vi "Set Window Title.vi"(8 "error in (no error)":errorcluster, 11 "Actor in":refnum<class "Actor.lvclass">) -> (0 "error out":errorcluster)   [LabVIEW 2020, in "RTAF.lvlib" / "Actor.lvclass"]
uses:
  Actor.lvclass
  Actor.lvclass/Actor.ctl
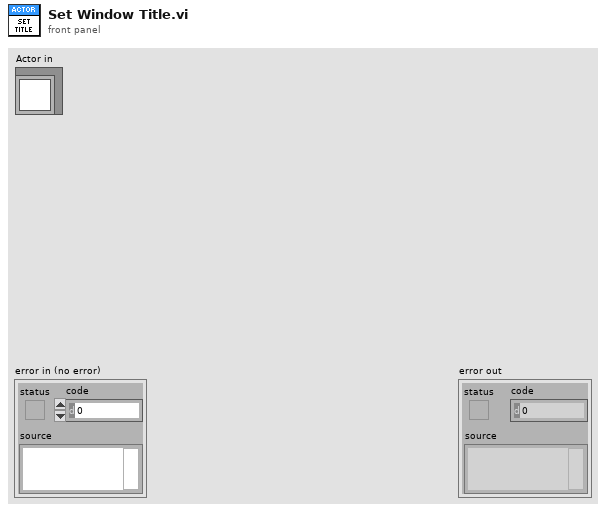
[diagram p1: front panel]
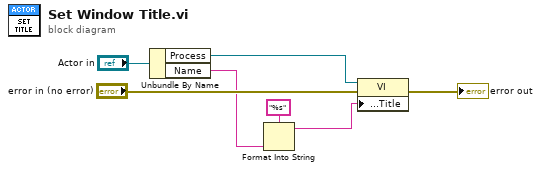
[diagram p0: block diagram]
diagram:
  n1 = Unbundle By Name("Actor in") -> ("Process"=w5:refnum<vi>, "Name"=w2:string)
  n2 = Format Into String(format string="%s", w2) -> (resulting string=w1:string)  [unwired: 2 in, 1 out]
  n3 = property class="VI"(reference=w5, error in="error in (no error)", "Front Panel.Title"=w1) -> (error out=→"error out":errorcluster)  [unwired: 1 out]
